vi "JSONconfig_VISAPowerSupplyArray.vi"(2 "error in (no error)":errorcluster, 3 "String":string, 4 "VISAPowerInfoInputArray":T1[](array[typedef])) -> (0 "error out":errorcluster, 1 "VISAPowerInfoOutputArray":T1[](array[typedef]))   [LabVIEW 2019]
uses:
  Controls/VISA_power_Control.ctl
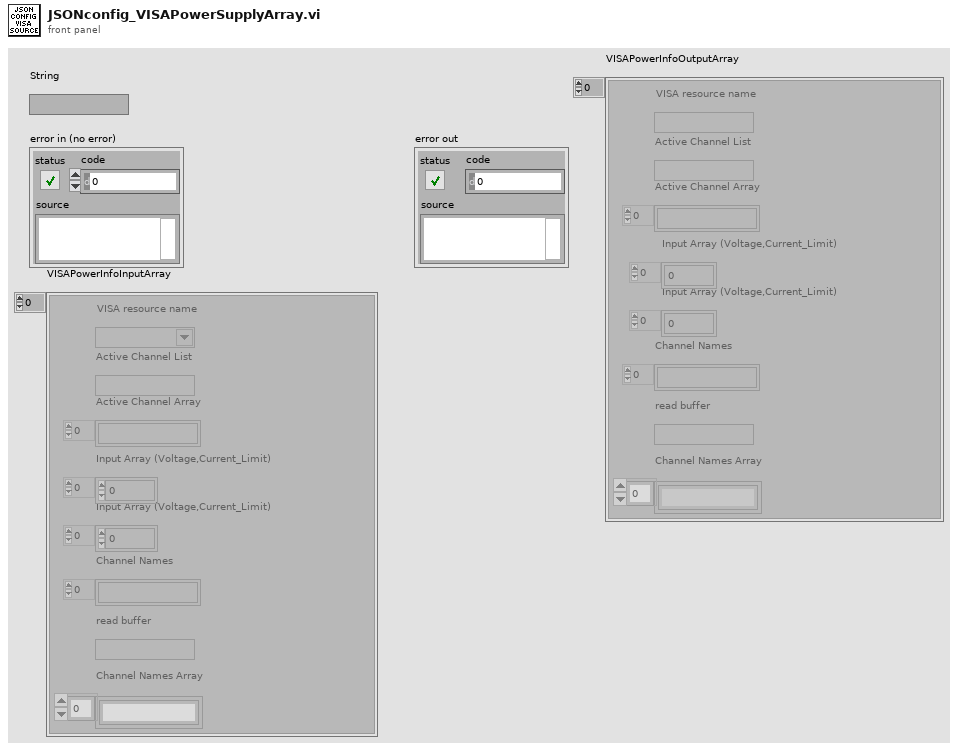
[diagram p1: front panel]
types:
  T1 = typedef "VISA_power_Control.ctl" = cluster{"VISA resource name":refnum<visa-resource-name>, "Active Channel List":string, "Active Channel Array":string[], "Input Array (Voltage,Current_Limit)":dbl[], "Input Array (Voltage,Current_Limit)":dbl[], "Channel Names":string[], "read buffer":string, "Channel Names Array":string[]}
  T2 = cluster{"VISA_Supply_Number":dbl, "VISA_Supply_Array":cluster{"VISA_GPIB_address":dbl, "combination_OFF_SER_PAR":string, "paralleled_channels_NA_ALL_I1+I2_I2+I3":string, "voltage_array_CH_1_2_3":dbl[], "current_array_CH_1_2_3":dbl[], "channel_names":string[]}[]}
  T3 = cluster{"VISA_GPIB_address":dbl, "combination_OFF_SER_PAR":string, "paralleled_channels_NA_ALL_I1+I2_I2+I3":string, "voltage_array_CH_1_2_3":dbl[], "current_array_CH_1_2_3":dbl[], "channel_names":string[]}[]
  T4 = cluster{"VISA resource name out":refnum<visa-resource-name>, "String List":string, "callable channels":string[], "voltage current double array":dbl[], "voltage current double array":dbl[], "channel_names":string[], "read buffer":string, "channel_names":string[]}
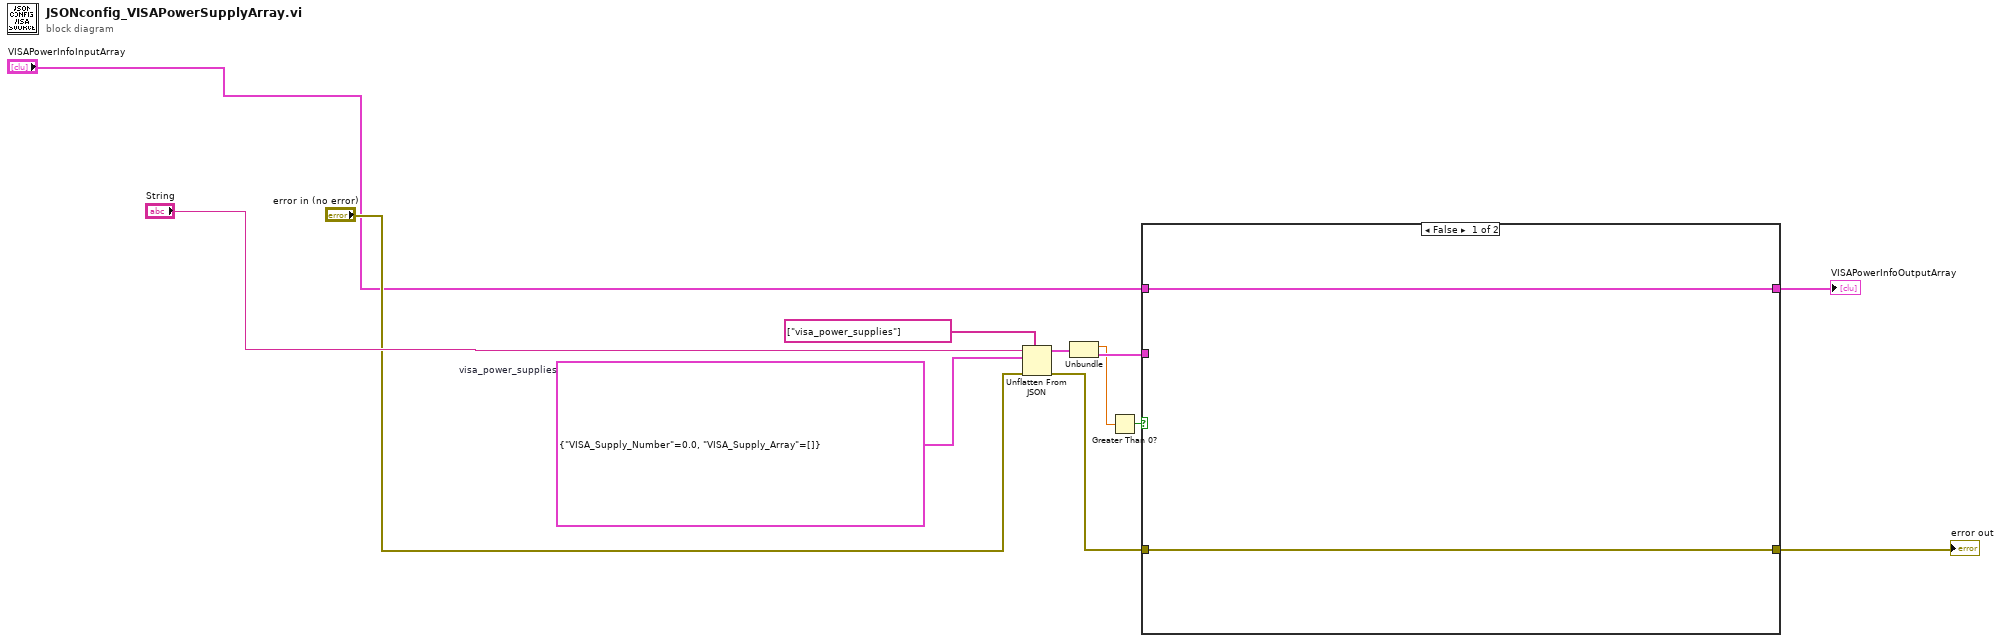
[diagram p0: block diagram]
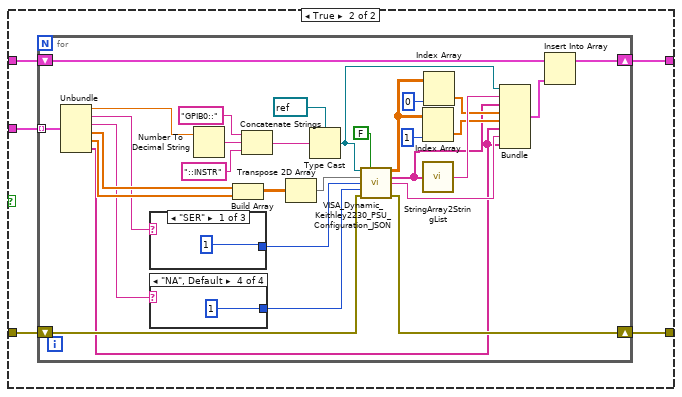
[diagram p2: hidden frame]
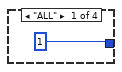
[diagram p3: hidden frame]
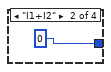
[diagram p4: hidden frame]
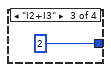
[diagram p5: hidden frame]
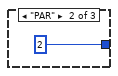
[diagram p6: hidden frame]
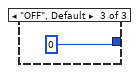
[diagram p7: hidden frame]
diagram:
  w10 = T2 {"VISA_Supply_Number"=0.0, "VISA_Supply_Array"=[]}  # visa_power_supplies
  n1 = Unflatten From JSON(path=string[] ["visa_power_supplies"], JSON string="String", type and defaults=w10, error in (no error)="error in (no error)") -> (value=w8:T2, error out=w9:errorcluster)  [unwired: 3 in]
  n2 = Unbundle(w8) -> ("VISA_Supply_Number"=w1:dbl, "VISA_Supply_Array"=w11:T3)
  n3 = Greater Than 0?(x=w1) -> (x > 0?=w2:bool)
  n4 = case shown="False" w2 {
    tunnel: [w13 w19] -> w12
    tunnel: w11 -> [_ w18]
    tunnel: w9 -> [w13 w17]
    tunnel: "VISAPowerInfoInputArray" -> [w14 w16]
    tunnel: [w14 w15] -> w3
    frame False {
    }
    frame True {
      n5 = for {
        shift-right: [w35] -> w19
        shift-left: w17 -> [w40]
        shift-right: [w23] -> w15
        shift-left: w16 -> [w20]
        tunnel: w18 -> [w24] mode=indexing
        n6 = Unbundle(w24) -> ("VISA_GPIB_address"=w26:dbl, "combination_OFF_SER_PAR"=w39:string, "paralleled_channels_NA_ALL_I1+I2_I2+I3"=w38:string, "voltage_array_CH_1_2_3"=w44:dbl[], "current_array_CH_1_2_3"=w43:dbl[], "channel_names"=w22:string[])
        n7 = case shown="\"SER\"" w39 {
          tunnel: [u16 1 u16 2 u16 0] -> w36
          frame "SER" {
          }
          frame "PAR" {
          }
          frame "OFF", Default {
          }
        }
        n8 = case shown="\"NA\", Default" w38 {
          tunnel: [u16 1 u16 0 u16 2 u16 1] -> w37
          frame "ALL" {
          }
          frame "I1+I2" {
          }
          frame "I2+I3" {
          }
          frame "NA", Default {
          }
        }
        n9 = Number To Decimal String(number=w26) -> (decimal integer string=w49:string)  [unwired: 1 in]
        n10 = Build Array(w44, w43) -> (w42:dbl[][])
        n11 = Concatenate Strings("GPIB0::" ("string"), w49, "::INSTR" ("string")) -> (w47:string)
        n12 = Transpose 2D Array(2D array=w42) -> (transposed array=w41:dbl[][])
        n13 = Type Cast(type=refnum<visa-resource-name> refnum ("VISA resource name out"), x=w47) -> (*(type *) &x=w31:refnum<visa-resource-name>)
        n14 = call "VISA_Dynamic_Keithley2230_PSU_Configuration_JSON.vi"("VISA resource name"=w31, "POWER STATUS IN"=FALSE, "Input Array (Voltage,Current_Limit)"=w41, "Combination Scheme"=w36, "Which Channels to Parallelize"=w37, "error in"=w40) -> ("voltage current double array"=w34:dbl[][], "callable channels"=w27:string[], "read buffer"=w25:string, "error out"=w35:errorcluster)  [unwired: 5 in, 1 out]
        n15 = Index Array(array=w34, index (col)=1 ("disabled index (col)")) -> (element=w28:dbl[])  [unwired: 1 in]
        n16 = call "StringArray2StringList.vi"("String Array"=w27) -> ("String List"=w30:string)
        n17 = Index Array(array=w34, index (col)=0 ("disabled index (col)")) -> (element=w29:dbl[])  [unwired: 1 in]
        n18 = Bundle("VISA resource name out"=w31, "String List"=w30, "callable channels"=w27, "voltage current double array"=w29, "voltage current double array"=w28, "channel_names"=w22, "read buffer"=w25, "channel_names"=w22) -> (w21:T4)  [unwired: 1 in]
        n19 = Insert Into Array(array=w20, new element=w21) -> (w23:T1[])  [unwired: 1 in]
      }
    }
  }
  "error out" <- w12
  "VISAPowerInfoOutputArray" <- w3
